vi "MotorSelect.vi"(3 "Motor":string="PI1-SHUTTER", 9 "error in (no error)":errorcluster) -> (0 "Motor out":string="PI1-SHUTTER", 6 "error out":errorcluster)   [LabVIEW 2009]
uses:
  Controls/MotorCommand.ctl
  Controls/MotorCommandBasic.ctl
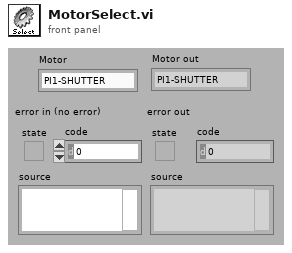
[diagram p1: front panel]
types:
  T1 = typedef "MotorCommandBasic.ctl" = enum16{"SELECT", "MOVE", "PREMOVE", "TURBO", "POS", "NAMED", "INIT", "STOP", "OFF", "SPEED", "QUIT"}
  T2 = typedef "MotorCommand.ctl" = cluster{"Motor":string, "Command":T1, "Movement":i32, "Name":string, "Param":cluster{"VMIN":i32, "VMAX":i32, "ACC":i32}, "Ok?":refnum<k4>, "Go!":refnum<k4>}
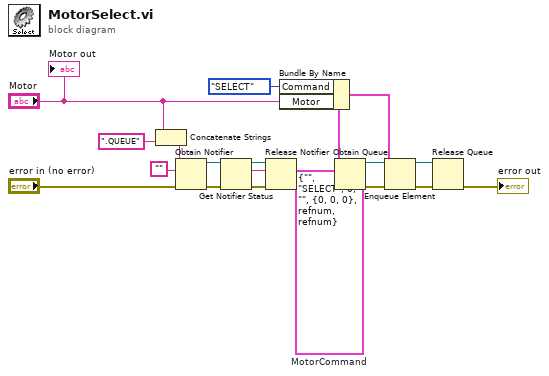
[diagram p0: block diagram]
diagram:
  w17 = T2 {"Motor"="", "Command"=enum."SELECT", "Movement"=0, "Name"="", "Param"={"VMIN"=0, "VMAX"=0, "ACC"=0}, "Ok?"=refnum, "Go!"=refnum}  # MotorCommand
  n1 = Concatenate Strings("Motor", ".QUEUE") -> (w8:string)
  n2 = Obtain Notifier(name (unnamed)=w8, notification data type="", error in (no error)="error in (no error)") -> (notifier out=w9:refnum<notifier>, error out=w10:errorcluster)  [unwired: 1 in, 1 out]
  n3 = Get Notifier Status(notifier=w9, error in (no error)=w10) -> (notifier out=w12:refnum<notifier>, current notification=w5:string, error out=w13:errorcluster)  [unwired: 2 out]
  n4 = Release Notifier(notifier=w12, error in (no error)=w13) -> (error out=w6:errorcluster)  [unwired: 3 out]
  n5 = Bundle By Name(cluster=w17, "Command"=MotorCommandBasic."SELECT", "Motor"="Motor") -> (w16:T2)
  n6 = Obtain Queue(name (unnamed)=w5, element data type=w17, error in (no error)=w6) -> (queue out=w19:refnum<queue>, error out=w18:errorcluster)  [unwired: 2 in, 1 out]
  n7 = Enqueue Element(queue=w19, element=w16, error in (no error)=w18) -> (queue out=w14:refnum<queue>, error out=w15:errorcluster)  [unwired: 2 out]
  n8 = Release Queue(queue=w14, error in (no error)=w15) -> (error out=→"error out":errorcluster)  [unwired: 3 out]
  "Motor out" <- "Motor"
